vi "Check3DStringArrayForDuplicates.vi"(11 "String Array":string[][][](array[string])) -> (3 "duplicate string found?":bool)   [LabVIEW 2012]
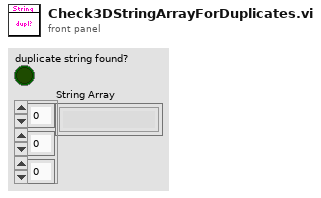
[diagram p1: front panel]
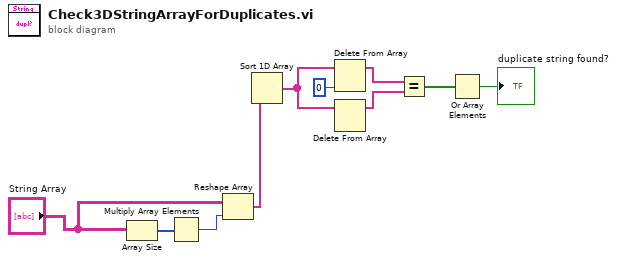
[diagram p0: block diagram]
diagram:
  n1 = Array Size(array="String Array") -> (size(s)=w4:i32[])
  n2 = Multiply Array Elements(1:w4) -> (0:w3:i32)
  n3 = Reshape Array("String Array", w3) -> (w2:string[])
  n4 = Sort 1D Array(array=w2) -> (sorted array=w10:string[])
  n5 = Delete From Array(array=w10, index=0) -> (array with subset deleted=w8:string[])  [unwired: 1 in, 1 out]
  n6 = Delete From Array(array=w10) -> (array with subset deleted=w7:string[])  [unwired: 2 in, 1 out]
  n7 = Equal?(x=w8, y=w7) -> (x = y?=w6:bool[])
  n8 = Or Array Elements(Boolean array=w6) -> (logical OR=→"duplicate string found?":bool)
